vi "Examen01.vi"() -> ()   [LabVIEW 2020]
uses:
  <vilib>/numeric/Random Number (Range) U64.vi
  <vilib>/numeric/sub_Random U32.vi
panel:
  out "Histeresis":bool
  out "Contador":dbl
  in  "stop":bool
  out "Tabla Excel":string[][](array[string])
  out "rango":bool
  in  "Limit Min":dbl
  in  "Limit Max":dbl
  out "Grafica (Randoms)":cluster{"number":u64, dbl}(graph)
  out "numero random":u64
  # "Rango:"
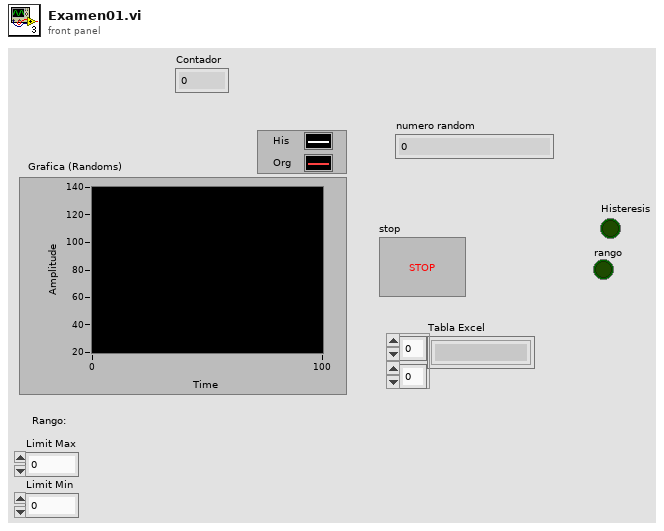
[diagram p1: front panel]
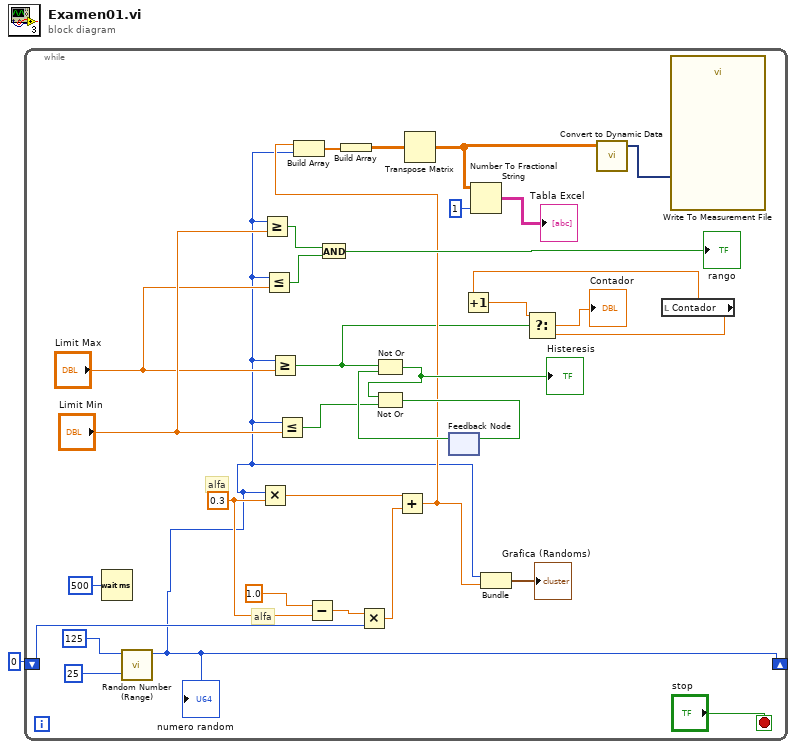
[diagram p0: block diagram]
diagram:
  n1 = while {
    shift-right: [w2] -> _
    shift-left: 0 -> [w25]
    stop <- "stop" stop-if-true
    w29 = 0.3 ("y")
    # "alfa"
    # "alfa"
    n2 = Wait (ms)(milliseconds to wait=u32 500) -> ()  [unwired: 1 out]
    n3 = call-poly <vilib>:"Random Number (Range).vi"("lower bound (0)"=u64 25, "upper bound (100)"=u64 125) -> ("number"=w2:u64)  [unwired: 9 in]
    "numero random" <- w2
    n4 = Multiply(x=w2, y=w29) -> (x*y=w28:dbl)
    n5 = Greater Or Equal?(x=w2, y="Limit Min") -> (x >= y?=w19:bool)
    n6 = Less Or Equal?(x=w2, y="Limit Max") -> (x <= y?=w18:bool)
    n7 = Greater Or Equal?(x=w2, y="Limit Max") -> (x >= y?=w3:bool)
    n8 = Less Or Equal?(x=w2, y="Limit Min") -> (x <= y?=w20:bool)
    n9 = Subtract(x=1.0, y=w29) -> (x-y=w26:dbl)
    n10 = And(x=w19, y=w18) -> (x .and. y?=→"rango":bool)
    n11 = Multiply(x=w26, y=w25) -> (x*y=w27:dbl)
    n12 = Add(x=w28, y=w27) -> (x+y=w13:dbl)
    n13 = Build Array(w13, w2) -> (w12:dbl[])
    n14 = Build Array(w12) -> (w11:dbl[][])
    n15 = Transpose Matrix(1:w11) -> (0:w15:dbl[][])
    n16 = feedback #1() -> (w23:bool)  [unwired: 1 in]
    n17 = Not Or(1:w23, 2:w3) -> (0:w21:bool)
    "Histeresis" <- w21
    n18 = Not Or(1:w20, 2:w21) -> (0:w22:bool)
    n19 = feedback-in #1(w22) -> ()
    n20 = Number To Fractional String(number=w15, precision (6)=i16 1) -> (F-format string=→"Tabla Excel":string[][])  [unwired: 2 in]
    n21 = Bundle("number"=w2, w13) -> (→"Grafica (Randoms)":cluster{"number":u64, dbl})  [unwired: 1 in]
    n22 = call "Convert to Dynamic Data"("2D Array"=w15) -> ("Dynamic Data Type"=w16:dynamicdata)  [unwired: 3 in]
    n23 = local read "Contador"() -> (w4:dbl)
    n24 = Increment(x=w4) -> (x+1=w6:dbl)
    n25 = Select(t=w6, s=w3, f=w4) -> (s? t:f=→"Contador":dbl)
    n26 = call "Write To Measurement File"("Signals"=w16) -> ()  [unwired: 16 in, 3 out]
  }
